vi "PDF Welding.vi"(0 "configuration file path":path caption="配置文件的路径", 1 "PDF Welding msic inf":T1) -> ()   [LabVIEW 2014]
uses:
  Ctl.xio/PDF Welding msic ctl.ctl
  SubVIS.xio/DataSocket/DataSocket_Tags.ctl
  Ctl.xio/part type.ctl
  SubVIS.xio/Creat Write List VI's/DefCtrl/Station.ctl
  SubVIS.xio/DataSocket/Write PLC Vars/Write Bool Var in.vi
  <vilib>/Utility/file.llb/Read From Spreadsheet File (string).vi
  SubVIS.xio/DataSocket/Write PLC Vars/Write String Var in.vi
  SubVIS.xio/DataSocket/Read PLC Vars/Read Bool Var.vi
  SubVIS.xio/DataSocket/Read PLC Vars/Read U32 Var.vi
  SubVIS.xio/DataSocket/Write PLC Vars/Write Dbl Var in.vi
  SubVIS.xio/Hopper car inf/Curing inf.vi
panel:
  in  "SQL information":string
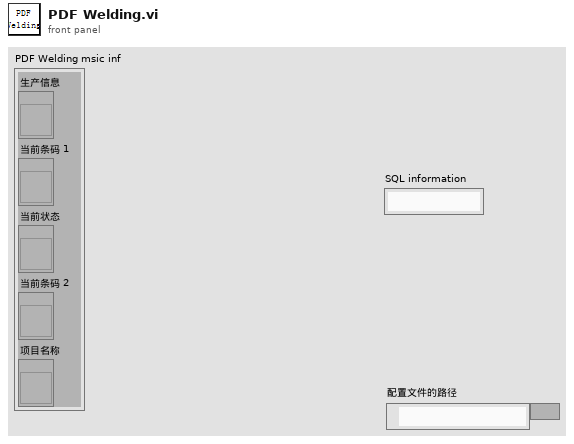
[diagram p1: front panel]
types:
  T1 = cluster{"生产信息":refnum<vi>, "当前条码 1":refnum<vi>, "当前状态":refnum<vi>, "当前条码 2":refnum<vi>, "项目名称":refnum<vi>}
  T2 = typedef "Station.ctl" = enum16{"粗切工位", "热处理工位", "精切工位", "PDF焊接工位", "打凹点预载力工位", "收卷工位", "EOL工位"}
  T3 = typedef "PDF Welding msic ctl.ctl" = cluster{"configuration file path":path, "DsOut":T4[], "Hopper car information":cluster{"Hopper car code":string, "Hopper car No":string, "plate No":string}, "pallet.produced number":i32, "SQL information":string, "Serial number":i32, "database path":path, "PDF Welding msic inf":cluster{"生产信息":refnum<vi>, "当前条码 1":refnum<vi>, "当前状态":refnum<vi>, "当前条码 2":refnum<vi>, "项目名称":refnum<vi>}, "Heating process parameters":cluster{"heating start":string, "heating finish":string, "Heating time use":u32}, "part type":T5, "Inlet temperature database":string[], "Outlet temperature database":string[], "Inlet temperature buffer":i32[], "Outlet temperature buffer":i32[], "PDF start time":string, "PDF finish time":string, "BarCode1":string, "BarCode2":string, "scanner resource name out":refnum<visa-resource-name>, "scanner coms or ip":string, "Outlet pressure buffer":i32[], "Outlet pressure database":string[], "scanner ip ID":refnum<k5>}
  T4 = typedef "DataSocket_Tags.ctl" = cluster{"Ds ID":refnum<k13>, "Tag":string}
  T5 = typedef "part type.ctl" = cluster{"项目号":string, "物料代码":string, "零件号":string, "供应商编码":string, "产线编码":string, "客户代码":string, "颜色代码":string, "托盘上限":i32, "加热温度":string, "加热时长":string, "EOL Stations":string}
  T6 = cluster{"Hopper car code":string, "Hopper car No":string, "plate No":string}
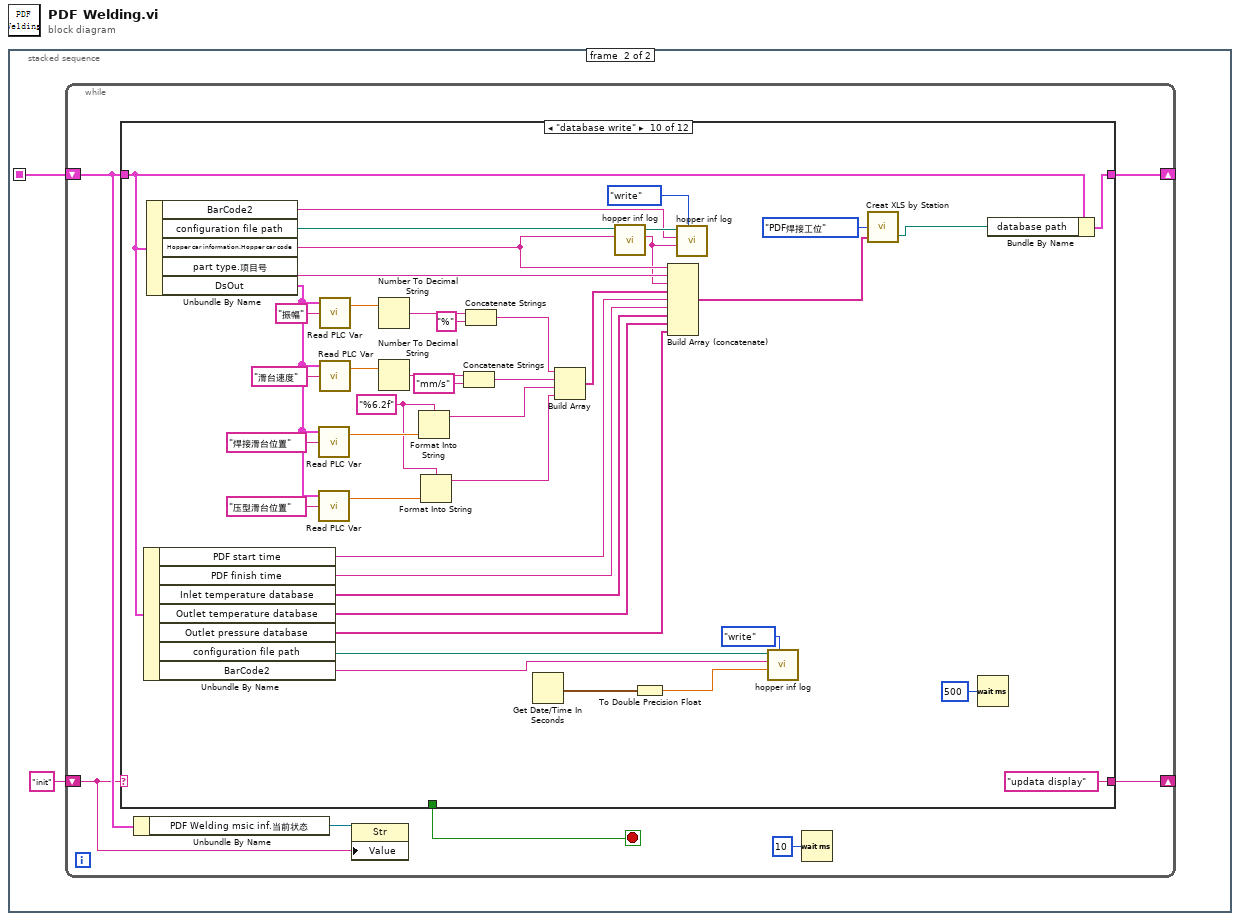
[diagram p0: block diagram]
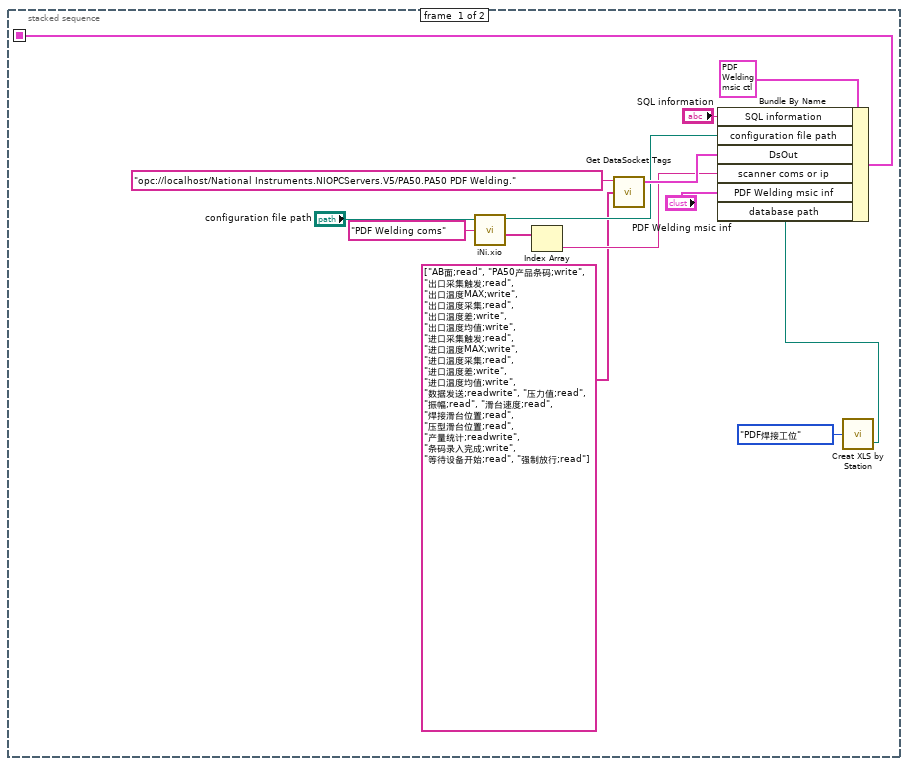
[diagram p2: hidden frame]
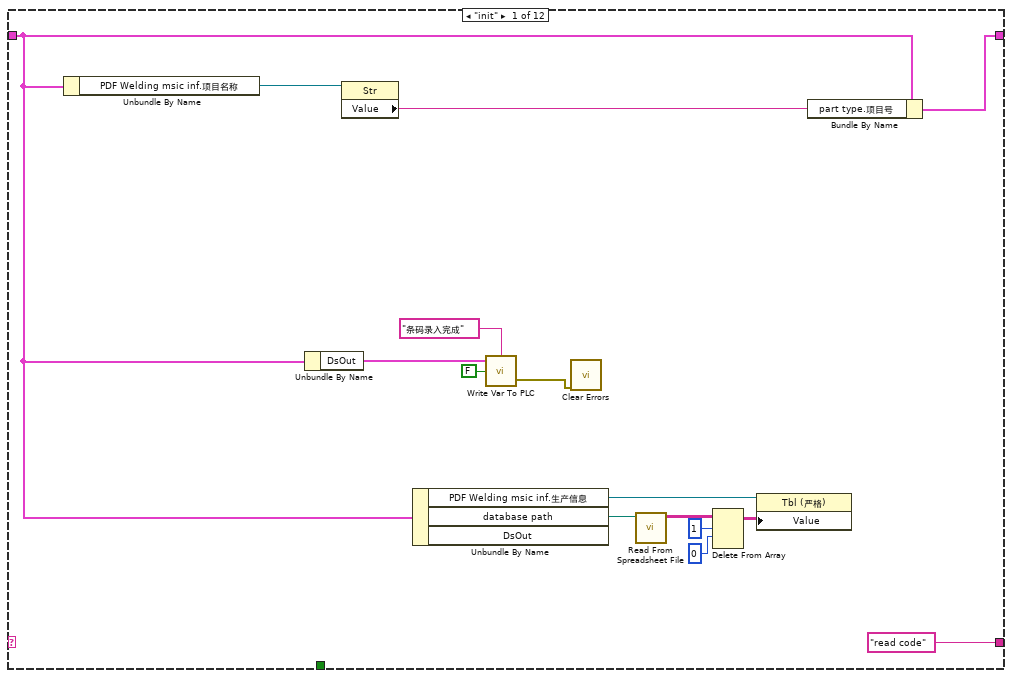
[diagram p3: hidden frame]
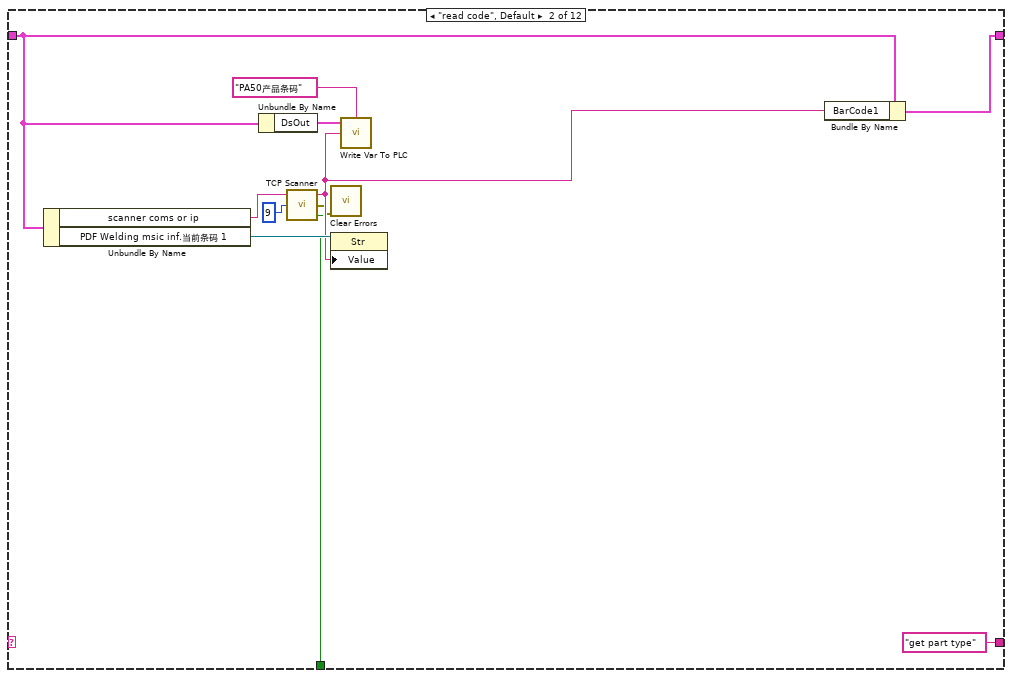
[diagram p4: hidden frame]
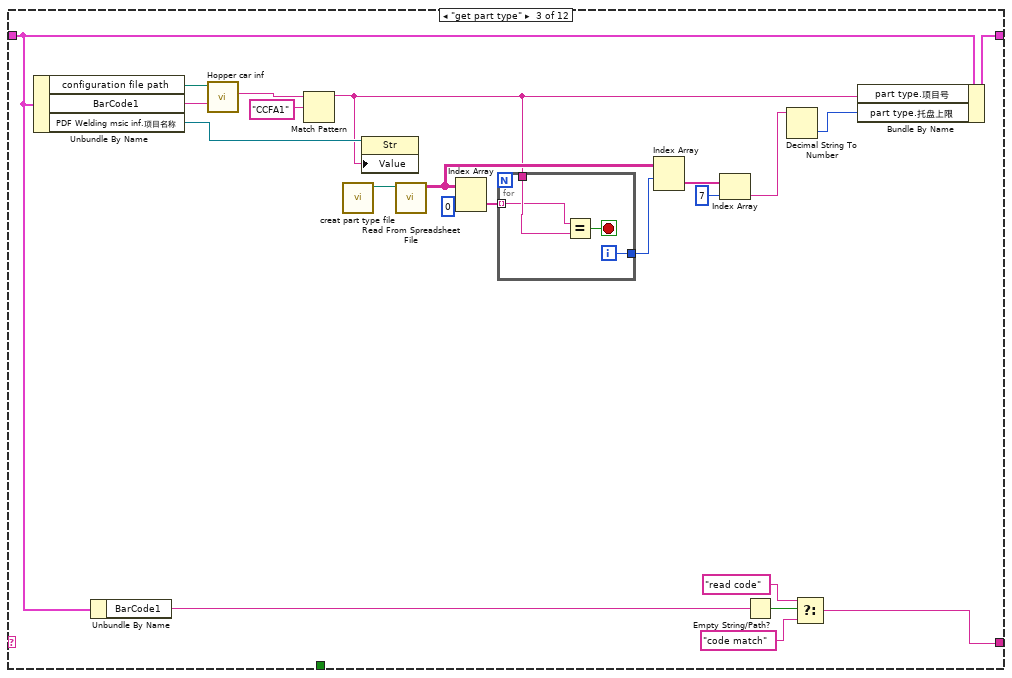
[diagram p5: hidden frame]
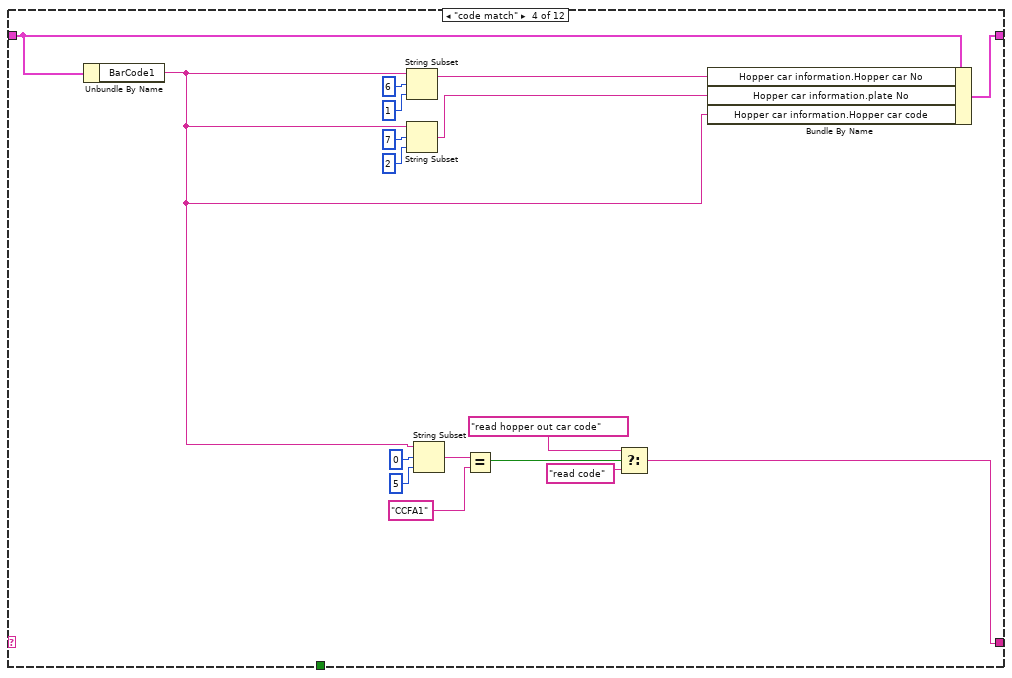
[diagram p6: hidden frame]
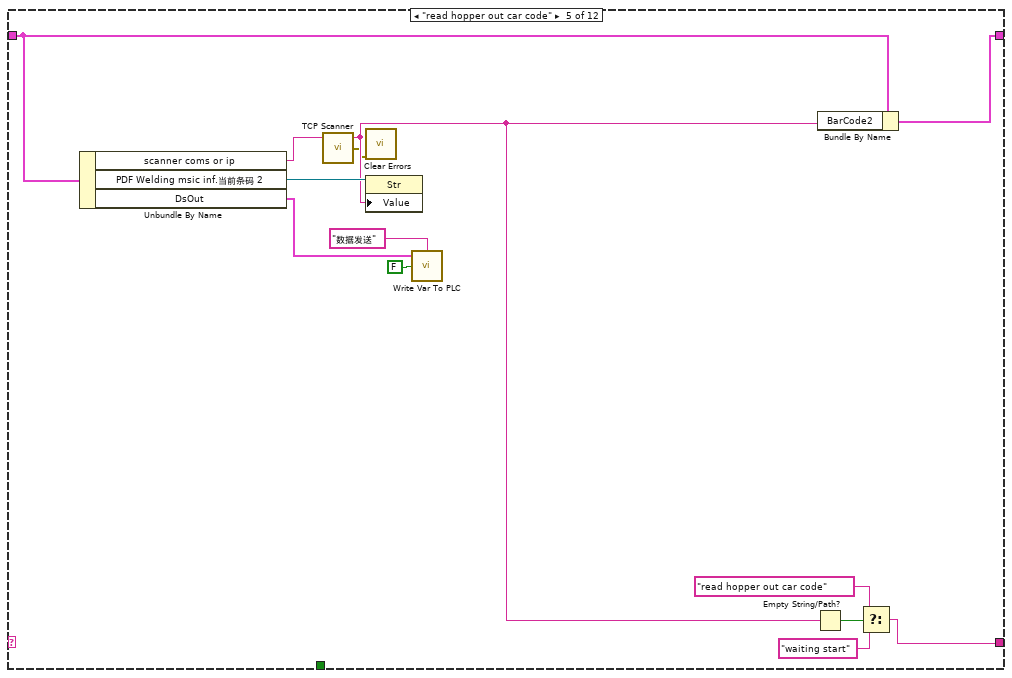
[diagram p7: hidden frame]
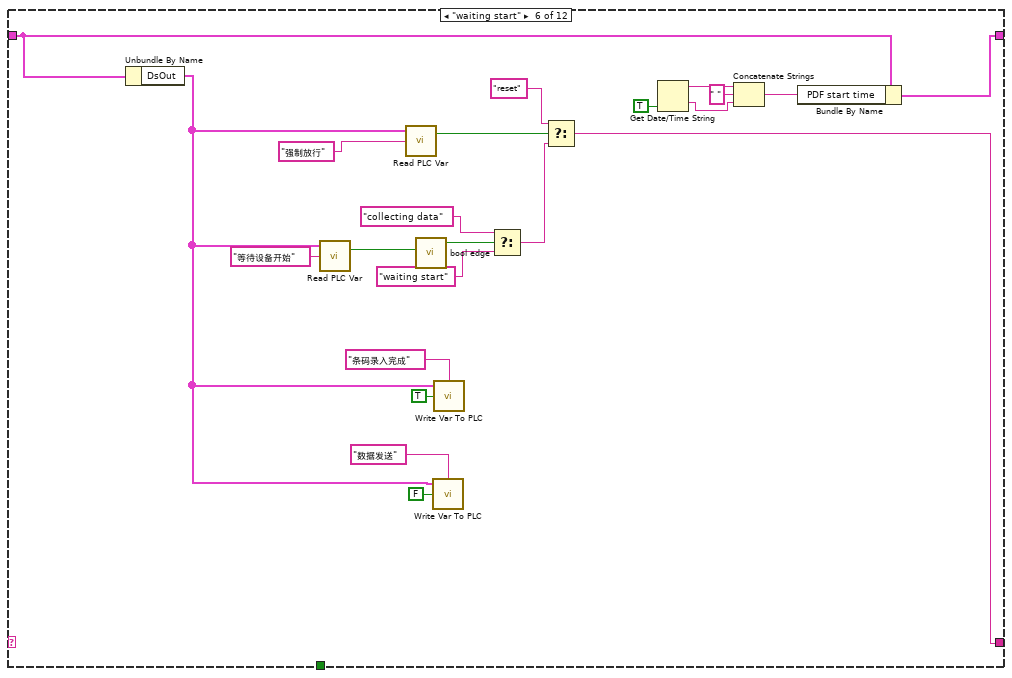
[diagram p8: hidden frame]
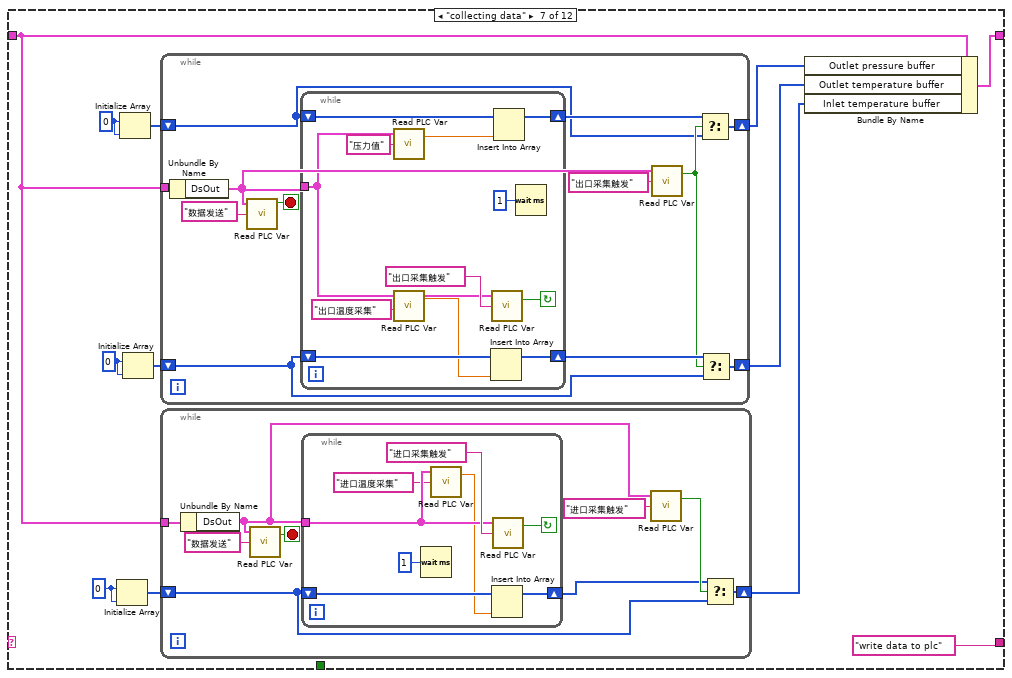
[diagram p9: hidden frame]
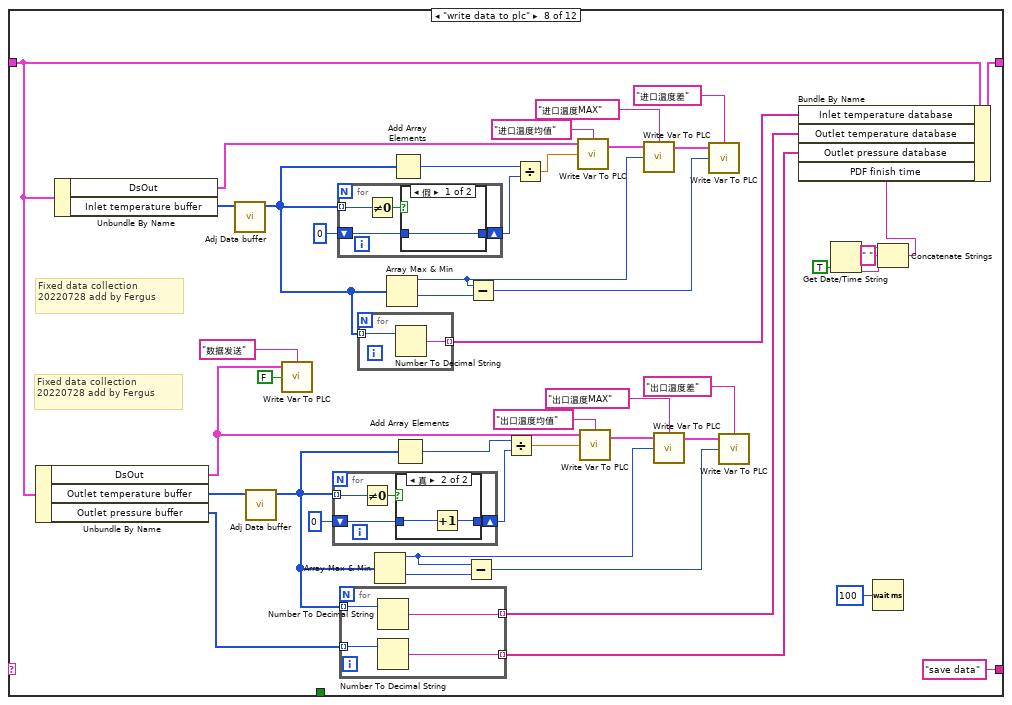
[diagram p10: hidden frame]
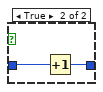
[diagram p12: hidden frame]
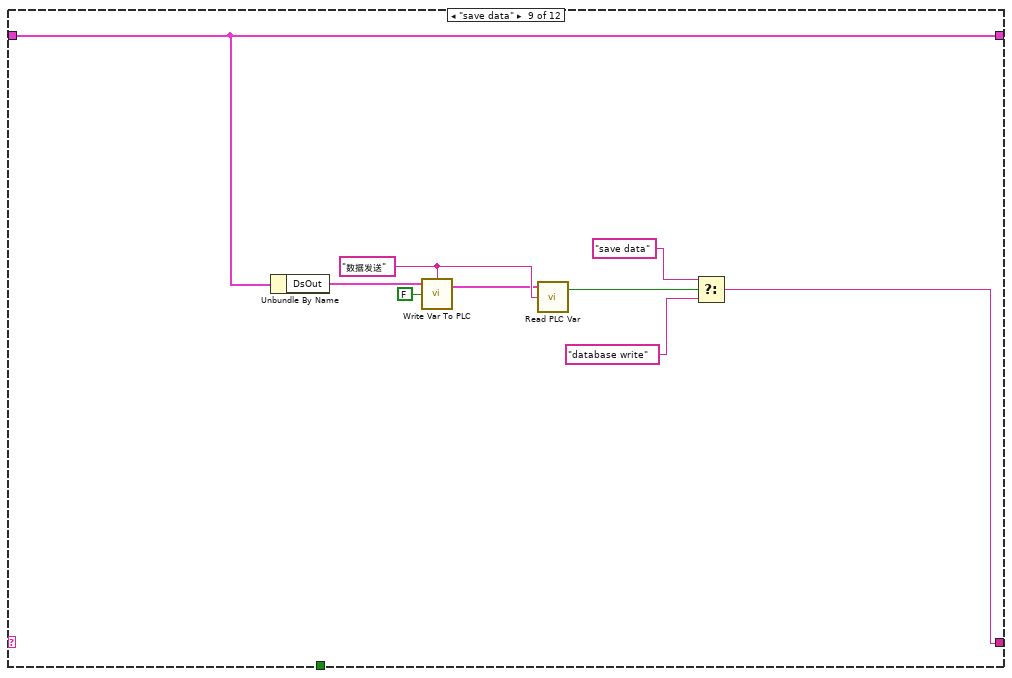
[diagram p13: hidden frame]
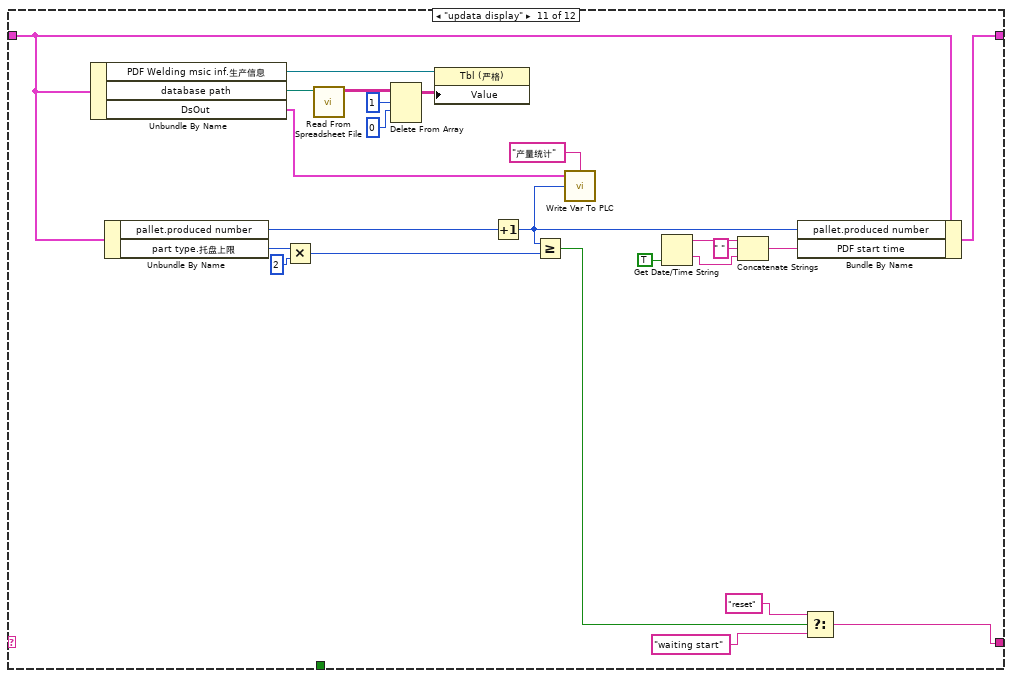
[diagram p14: hidden frame]
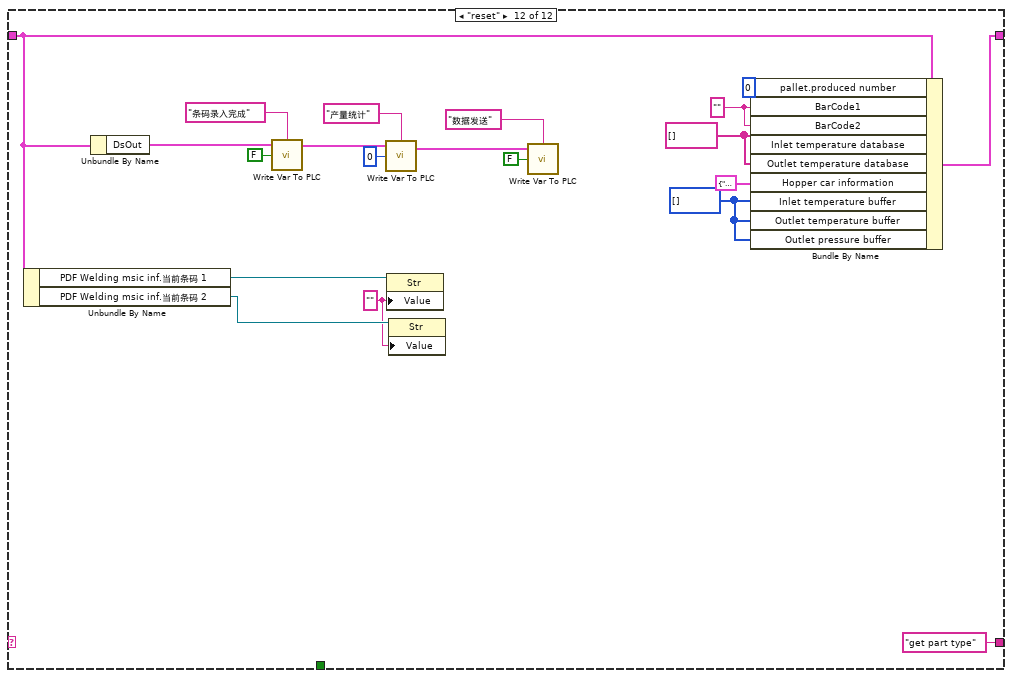
[diagram p15: hidden frame]
diagram:
  n1 = stacked-sequence {
    seq-local: [w3 _] -> [_ w15]
    frame #0 {
      n2 = call "iNi.xio.vi"("configuration file path"="configuration file path", "Sections"="PDF Welding coms") -> ("configuration file path"=w13:path, "Values"=w11:string[])  [unwired: 1 in, 3 out]
      n3 = Index Array(array=w11) -> (element=w10:string)  [unwired: 1 in]
      n4 = call "Get DataSocket Tags.vi"("All Tags"=string[] ["AB面;read", "PA50产品条码;write", "出口采集触发;read", "出口温度MAX;write", "出口温度采集;read", "出口温度差;write", "出口温度均值;write", "进口采集触发;read", "进口温度MAX;write", "进口温度采集;read", "进口温度差;write", "进口温度均值;write", "数据发送;readwrite", "压力值;read", "振幅;read", "滑台速度;read", "焊接滑台位置;read", "压型滑台位置;read", "产量统计;readwrite", "条码录入完成;write", "等待设备开始;read", "强制放行;read"], "URL"="opc://localhost/National Instruments.NIOPCServers.V5/PA50.PA50 PDF Welding.") -> ("DsOut"=w14:T4[])  [unwired: 3 in]
      n5 = call "Creat XLS by Station.vi"("staiton"=Station."PDF焊接工位") -> ("new file path (Not A Path if cancelled)"=w1:path)  [unwired: 5 in]
      n6 = Bundle By Name(cluster=T3 {"configuration file path"=path "", "DsOut"=[], "Hopper car information"={"Hopper car code"="", "Hopper car No"="", "plate No"=""}, "pallet.produced number"=0, "SQL information"="", "Serial number"=0, "database path"=path "", "PDF Welding msic inf"={"生产信息"=refnum, "当前条码 1"=refnum, "当前状态"=refnum, "当前条码 2"=refnum, "项目名称"=refnum}, "Heating process parameters"={"heating start"="", "heating finish"="", "Heating time use"=0}, "part type"={"项目号"="", "物料代码"="", "零件号"="", "供应商编码"="", "产线编码"="", "客户代码"="", "颜色代码"="", "托盘上限"=0, "加热温度"="", "加热时长"="", "EOL Stations"=""}, "Inlet temperature database"=[], "Outlet temperature database"=[], "Inlet temperature buffer"=[], "Outlet temperature buffer"=[], "PDF start time"="", "PDF finish time"="", "BarCode1"="", "BarCode2"="", "scanner resource name out"="", "scanner coms or ip"="", "Outlet pressure buffer"=[], "Outlet pressure database"=[], "scanner ip ID"=refnum} ("PDF Welding msic ctl"), "SQL information"="SQL information", "configuration file path"=w13, "DsOut"=w14, "scanner coms or ip"=w10, "PDF Welding msic inf"="PDF Welding msic inf", "database path"=w1) -> (w3:T3)
    }
    frame #1 {
      n7 = while {
        shift-right: [w23] -> _
        shift-left: w15 -> [w19]
        shift-right: [w22] -> _
        shift-left: "init" ("event") -> [w18]
        stop <- w17 stop-if-true
        n8 = case shown="\"database write\"" w18 {
          tunnel: w19 -> [w25 w46 w54 w78 w104 w108 w128 w196 w253 w295 w312 w331]
          tunnel: [w38 w49 w71 w86 w103 w106 w139 w197 w253 w296 w311 w340] -> w23
          tunnel: ["read code" "get part type" ("f") w58 w85 w97 w119 "write data to plc" ("f") "save data" ("f") w246 "updata display" ("f") w307 "get part type" ("f")] -> w22
          tunnel: [_ w39 _ _ _ _ _ _ _ _ _ _] -> w17
          frame "init" {
            n9 = Unbundle By Name(w25) -> ("PDF Welding msic inf.项目名称"=w37:refnum<vi>)
            n10 = Unbundle By Name(w25) -> ("DsOut"=w34:T4[])
            n11 = property class="Str"(reference=w37) -> ("Value"=w36:string)  [unwired: 1 in, 2 out]
            n12 = Unbundle By Name(w25) -> ("PDF Welding msic inf.生产信息"=w31:refnum<vi>, "database path"=w30:path)  [unwired: 1 out]
            n13 = call-poly "Write Var To PLC.vi"("Tag IN"="条码录入完成", "Bool Var in"=FALSE, "Ds PLCTags IN"=w34) -> ("error out"=w24:errorcluster)  [unwired: 1 in, 1 out]
            n14 = call <vilib>:"Clear Errors.vi"("error in (no error)"=w24) -> ()  [unwired: 5 in, 2 out]
            n15 = call-poly <vilib>:"Read From Spreadsheet File.vi"("file path (dialog if empty)"=w30) -> ("all rows"=w29:string[][])  [unwired: 6 in, 4 out]
            n16 = Delete From Array(array=w29, length=1 ("长度"), index (row)=0 ("索引 (行)")) -> (array with subset deleted=w26:string[][])  [unwired: 1 in, 1 out]
            n17 = property class="Tbl (严格)"(reference=w31, "Value"=w26) -> ()  [unwired: 1 in, 2 out]
            n18 = Bundle By Name(cluster=w25, "part type.项目号"=w36) -> (w38:T3)
          }
          frame "read code", Default {
            n19 = Unbundle By Name(w46) -> ("scanner coms or ip"=w42:string, "PDF Welding msic inf.当前条码 1"=w48:refnum<vi>)
            n20 = Unbundle By Name(w46) -> ("DsOut"=w45:T4[])
            n21 = call "TCP Scanner.vi"("byte of read(9)"=9 ("读取的字节"), "ip"=w42) -> ("status"=w39:bool, "错误输出"=w40:errorcluster, "Barcode"=w44:string)  [unwired: 1 in]
            n22 = call <vilib>:"Clear Errors.vi"("error in (no error)"=w40) -> ()  [unwired: 5 in, 2 out]
            n23 = property class="Str"(reference=w48, "Value"=w44) -> ()  [unwired: 1 in, 2 out]
            n24 = call-poly "Write Var To PLC.vi"("Tag IN"="PA50产品条码", "String Var in"=w44, "Ds PLCTags IN"=w45) -> ()  [unwired: 1 in, 2 out]
            n25 = Bundle By Name(cluster=w46, "BarCode1"=w44) -> (w49:T3)
          }
          frame "get part type" {
            n26 = Unbundle By Name(w54) -> ("configuration file path"=w56:path, "BarCode1"=w55:string, "PDF Welding msic inf.项目名称"=w53:refnum<vi>)
            n27 = Unbundle By Name(w54) -> ("BarCode1"=w57:string)
            n28 = call "Hopper car inf.vi"("key"=w55, "path in"=w56) -> ("value out"=w52:string)  [unwired: 8 in, 1 out]
            n29 = Match Pattern(string=w52, regular expression="CCFA1" ("正则表达式")) -> (before substring=w50:string)  [unwired: 1 in, 3 out]
            n30 = call "creat part type file.vi"() -> ("new file path (Not A Path if cancelled)"=w62:path)  [unwired: 11 in]
            n31 = property class="Str"(reference=w53, "Value"=w50) -> ()  [unwired: 1 in, 2 out]
            n32 = call-poly <vilib>:"Read From Spreadsheet File.vi"("file path (dialog if empty)"=w62) -> ("all rows"=w67:string[][])  [unwired: 6 in, 4 out]
            n33 = Index Array(array=w67, index (col)=0 ("禁用的索引 (列)")) -> (element=w69:string[])  [unwired: 1 in]
            n34 = for {
              tunnel: w69 -> [w72] mode=indexing
              tunnel: [w74] -> w66
              tunnel: w50 -> [w73]
              i -> [w74]
              stop <- w75 stop-if-true
              n35 = Equal?(x=w72, y=w73) -> (x = y?=w75:bool)
            }
            n36 = Index Array(array=w67, index (row)=w66) -> (element=w65:string[])  [unwired: 1 in]
            n37 = Index Array(array=w65, index=7 ("索引")) -> (element=w64:string)
            n38 = Empty String/Path?(string/path=w57) -> (empty?=w61:bool)
            n39 = Decimal String To Number(string=w64) -> (number=w63:i32)  [unwired: 2 in, 1 out]
            n40 = Select(t="read code", s=w61, f="code match") -> (s? t:f=w58:string)
            n41 = Bundle By Name(cluster=w54, "part type.项目号"=w50, "part type.托盘上限"=w63) -> (w71:T3)
          }
          frame "code match" {
            n42 = Unbundle By Name(w78) -> ("BarCode1"=w77:string)
            n43 = String Subset(string=w77, offset (0)=6 ("偏移量(0)"), length (rest)=1 ("长度（剩余）")) -> (substring=w80:string)
            n44 = String Subset(string=w77, offset (0)=7 ("偏移量(0)"), length (rest)=2 ("长度（剩余）")) -> (substring=w81:string)
            n45 = String Subset(string=w77, offset (0)=0 ("偏移量(0)"), length (rest)=5 ("长度（剩余）")) -> (substring=w82:string)
            n46 = Equal?(x=w82, y="CCFA1") -> (x = y?=w76:bool)
            n47 = Select(t="read hopper out car code" ("event"), s=w76, f="read code" ("event")) -> (s? t:f=w85:string)
            n48 = Bundle By Name(cluster=w78, "Hopper car information.Hopper car No"=w80, "Hopper car information.plate No"=w81, "Hopper car information.Hopper car code"=w77) -> (w86:T3)
          }
          frame "read hopper out car code" {
            n49 = Unbundle By Name(w104) -> ("scanner coms or ip"=w105:string, "PDF Welding msic inf.当前条码 2"=w102:refnum<vi>, "DsOut"=w93:T4[])
            n50 = call "TCP Scanner.vi"("ip"=w105) -> ("错误输出"=w96:errorcluster, "Barcode"=w98:string)  [unwired: 2 in, 1 out]
            n51 = call <vilib>:"Clear Errors.vi"("error in (no error)"=w96) -> ()  [unwired: 5 in, 2 out]
            n52 = property class="Str"(reference=w102, "Value"=w98) -> ()  [unwired: 1 in, 2 out]
            n53 = call-poly "Write Var To PLC.vi"("Tag IN"="数据发送", "Bool Var in"=FALSE, "Ds PLCTags IN"=w93) -> ()  [unwired: 1 in, 2 out]
            n54 = Empty String/Path?(string/path=w98) -> (empty?=w101:bool)
            n55 = Bundle By Name(cluster=w104, "BarCode2"=w98) -> (w103:T3)
            n56 = Select(t="read hopper out car code" ("f"), s=w101, f="waiting start") -> (s? t:f=w97:string)
          }
          frame "waiting start" {
            n57 = Unbundle By Name(w108) -> ("DsOut"=w113:T4[])
            n58 = call-poly "Read PLC Var.vi"("Tag IN"="等待设备开始", "Ds PLCTags IN"=w113) -> ("Bool Var out"=w126:bool)  [unwired: 1 in, 1 out]
            n59 = call-poly "Read PLC Var.vi"("Tag IN"="强制放行", "Ds PLCTags IN"=w113) -> ("Bool Var out"=w121:bool)  [unwired: 1 in, 1 out]
            n60 = call "bool edge.vi"("bool in"=w126) -> ("false-true"=w125:bool)  [unwired: 6 in, 1 out]
            n61 = call-poly "Write Var To PLC.vi"("Tag IN"="数据发送", "Bool Var in"=FALSE, "Ds PLCTags IN"=w113) -> ()  [unwired: 1 in, 2 out]
            n62 = call-poly "Write Var To PLC.vi"("Tag IN"="条码录入完成", "Bool Var in"=TRUE, "Ds PLCTags IN"=w113) -> ()  [unwired: 1 in, 2 out]
            n63 = Select(t="collecting data" ("f"), s=w125, f="waiting start") -> (s? t:f=w120:string)
            n64 = Select(t="reset" ("f"), s=w121, f=w120) -> (s? t:f=w119:string)
            n65 = Get Date/Time String(want seconds? (F)=TRUE ("需要秒？(F)")) -> (date string=w112:string, time string=w110:string)  [unwired: 2 in]
            n66 = Concatenate Strings(w112, " " ("字符串"), w110) -> (w107:string)
            n67 = Bundle By Name(cluster=w108, "PDF start time"=w107) -> (w106:T3)
          }
          frame "collecting data" {
            w131 = 0 ("维数大小")
            w133 = 0 ("维数大小")
            w136 = 0 ("维数大小")
            n68 = Initialize Array(w133, w133) -> (w132:i32[])
            n69 = Initialize Array(w131, w131) -> (w130:i32[])
            n70 = Initialize Array(w136, w136) -> (w135:i32[])
            n71 = while {
              tunnel: w128 -> [w168]
              shift-right: [w161] -> w134
              shift-left: w135 -> [w162]
              shift-right: [w160] -> w129
              shift-left: w130 -> [w157]
              stop <- w166 stop-if-true
              n72 = Unbundle By Name(w168) -> ("DsOut"=w165:T4[])
              n73 = call-poly "Read PLC Var.vi"("Tag IN"="数据发送", "Ds PLCTags IN"=w165) -> ("Bool Var out"=w166:bool)  [unwired: 1 in, 1 out]
              n74 = while {
                tunnel: w165 -> [w173]
                shift-right: [w175] -> w163
                shift-left: w162 -> [w177]
                shift-right: [w169] -> w158
                shift-left: w157 -> [w170]
                stop <- w180 continue-if-true
                n75 = call-poly "Read PLC Var.vi"("Tag IN"="压力值", "Ds PLCTags IN"=w173) -> ("U32 Var out"=w171:dbl)  [unwired: 1 in, 1 out]
                n76 = call-poly "Read PLC Var.vi"("Tag IN"="出口温度采集", "Ds PLCTags IN"=w173) -> ("U32 Var out"=w176:dbl)  [unwired: 1 in, 1 out]
                n77 = Insert Into Array(array=w177, new element=w176) -> (w175:i32[])  [unwired: 1 in]
                n78 = call-poly "Read PLC Var.vi"("Tag IN"="出口采集触发", "Ds PLCTags IN"=w173) -> ("Bool Var out"=w180:bool)  [unwired: 1 in, 1 out]
                n79 = Insert Into Array(array=w170, new element=w171) -> (w169:i32[])  [unwired: 1 in]
                n80 = Wait (ms)(milliseconds to wait=u32 1 ("等待时间（毫秒）")) -> ()  [unwired: 1 out]
              }
              n81 = call-poly "Read PLC Var.vi"("Tag IN"="出口采集触发", "Ds PLCTags IN"=w165) -> ("Bool Var out"=w159:bool)  [unwired: 1 in, 1 out]
              n82 = Select(t=w158, s=w159, f=w157) -> (s? t:f=w160:i32[])
              n83 = Select(t=w163, s=w159, f=w162) -> (s? t:f=w161:i32[])
            }
            n84 = while {
              tunnel: w128 -> [w148]
              shift-right: [w143] -> w138
              shift-left: w132 -> [w140]
              stop <- w146 stop-if-true
              n85 = Unbundle By Name(w148) -> ("DsOut"=w145:T4[])
              n86 = call-poly "Read PLC Var.vi"("Tag IN"="数据发送", "Ds PLCTags IN"=w145) -> ("Bool Var out"=w146:bool)  [unwired: 1 in, 1 out]
              n87 = while {
                tunnel: w145 -> [w154]
                shift-right: [w150] -> w141
                shift-left: w140 -> [w152]
                stop <- w156 continue-if-true
                n88 = Wait (ms)(milliseconds to wait=u32 1 ("等待时间（毫秒）")) -> ()  [unwired: 1 out]
                n89 = call-poly "Read PLC Var.vi"("Tag IN"="进口温度采集", "Ds PLCTags IN"=w154) -> ("U32 Var out"=w151:dbl)  [unwired: 1 in, 1 out]
                n90 = Insert Into Array(array=w152, new element=w151) -> (w150:i32[])  [unwired: 1 in]
                n91 = call-poly "Read PLC Var.vi"("Tag IN"="进口采集触发", "Ds PLCTags IN"=w154) -> ("Bool Var out"=w156:bool)  [unwired: 1 in, 1 out]
              }
              n92 = call-poly "Read PLC Var.vi"("Tag IN"="进口采集触发", "Ds PLCTags IN"=w145) -> ("Bool Var out"=w142:bool)  [unwired: 1 in, 1 out]
              n93 = Select(t=w141, s=w142, f=w140) -> (s? t:f=w143:i32[])
            }
            n94 = Bundle By Name(cluster=w128, "Outlet pressure buffer"=w129, "Outlet temperature buffer"=w134, "Inlet temperature buffer"=w138) -> (w139:T3)
          }
          frame "write data to plc" {
            # "Fixed data collection\n20220728 add by Fergus"
            # "Fixed data collection\n20220728 add by Fergus"
            n95 = Unbundle By Name(w196) -> ("DsOut"=w193:T4[], "Outlet temperature buffer"=w182:i32[], "Outlet pressure buffer"=w187:i32[])
            n96 = Unbundle By Name(w196) -> ("DsOut"=w221:T4[], "Inlet temperature buffer"=w184:i32[])
            n97 = call "Adj Data buffer.vi"("data buffer"=w184) -> ("data buffer out"=w183:i32[])  [unwired: 10 in]
            n98 = call "Adj Data buffer.vi"("data buffer"=w182) -> ("data buffer out"=w181:i32[])  [unwired: 10 in]
            n99 = call-poly "Write Var To PLC.vi"("Tag IN"="数据发送", "Bool Var in"=FALSE, "Ds PLCTags IN"=w193) -> ()  [unwired: 1 in, 2 out]
            n100 = for {
              tunnel: w181 -> [w235] mode=indexing
              shift-right: [w232] -> w216
              shift-left: 0 -> [w233]
              n101 = Not Equal To 0?(x=w235) -> (x != 0?=w234:bool)
              n102 = case shown="真" w234 {
                tunnel: w233 -> [w236 w237]
                tunnel: [w236 w238] -> w232
                frame False {
                }
                frame True {
                  n103 = Increment(x=w237) -> (x+1=w238:i32)
                }
              }
            }
            n104 = for {
              tunnel: w183 -> [w242] mode=indexing
              shift-right: [w239] -> w223
              shift-left: 0 -> [w240]
              n105 = Not Equal To 0?(x=w242) -> (x != 0?=w241:bool)
              n106 = case shown="假" w241 {
                tunnel: w240 -> [w243 w244]
                tunnel: [w243 w245] -> w239
                frame False {
                }
                frame True {
                  n107 = Increment(x=w244) -> (x+1=w245:i32)
                }
              }
            }
            n108 = for {
              tunnel: w181 -> [w229] mode=indexing
              tunnel: [w227] -> w199 mode=indexing
              tunnel: w187 -> [w228] mode=indexing
              tunnel: [w226] -> w185 mode=indexing
              n109 = Number To Decimal String(number=w229) -> (decimal integer string=w227:string)  [unwired: 1 in]
              n110 = Number To Decimal String(number=w228) -> (decimal integer string=w226:string)  [unwired: 1 in]
            }
            n111 = for {
              tunnel: w183 -> [w231] mode=indexing
              tunnel: [w230] -> w200 mode=indexing
              n112 = Number To Decimal String(number=w231) -> (decimal integer string=w230:string)  [unwired: 1 in]
            }
            n113 = Array Max & Min(array=w181) -> (max value=w203:i32, min value=w202:i32)  [unwired: 2 out]
            n114 = Array Max & Min(array=w183) -> (max value=w211:i32, min value=w214:i32)  [unwired: 2 out]
            n115 = Add Array Elements(numeric array=w183) -> (sum=w222:i32)
            n116 = Add Array Elements(numeric array=w181) -> (sum=w217:i32)
            n117 = Subtract(x=w203, y=w202) -> (x-y=w201:i32)
            n118 = Subtract(x=w211, y=w214) -> (x-y=w208:i32)
            n119 = Divide(x=w217, y=w216) -> (x/y=w215:dbl)
            n120 = Divide(x=w222, y=w223) -> (x/y=w219:dbl)
            n121 = call-poly "Write Var To PLC.vi"("Tag IN"="进口温度均值", "Dbl Var in"=w219, "Ds PLCTags IN"=w221) -> ("Ds PLCTags OUT"=w213:T4[])  [unwired: 1 in, 1 out]
            n122 = call-poly "Write Var To PLC.vi"("Tag IN"="出口温度均值", "Dbl Var in"=w215, "Ds PLCTags IN"=w193) -> ("Ds PLCTags OUT"=w204:T4[])  [unwired: 1 in, 1 out]
            n123 = call-poly "Write Var To PLC.vi"("Tag IN"="进口温度MAX", "Dbl Var in"=w211, "Ds PLCTags IN"=w213) -> ("Ds PLCTags OUT"=w210:T4[])  [unwired: 1 in, 1 out]
            n124 = call-poly "Write Var To PLC.vi"("Tag IN"="出口温度MAX", "Dbl Var in"=w203, "Ds PLCTags IN"=w204) -> ("Ds PLCTags OUT"=w206:T4[])  [unwired: 1 in, 1 out]
            n125 = call-poly "Write Var To PLC.vi"("Tag IN"="进口温度差", "Dbl Var in"=w208, "Ds PLCTags IN"=w210) -> ()  [unwired: 1 in, 2 out]
            n126 = call-poly "Write Var To PLC.vi"("Tag IN"="出口温度差", "Dbl Var in"=w201, "Ds PLCTags IN"=w206) -> ()  [unwired: 1 in, 2 out]
            n127 = Get Date/Time String(want seconds? (F)=TRUE ("需要秒？(F)")) -> (date string=w192:string, time string=w190:string)  [unwired: 2 in]
            n128 = Wait (ms)(milliseconds to wait=u32 100 ("等待时间（毫秒）")) -> ()  [unwired: 1 out]
            n129 = Concatenate Strings(w192, " " ("字符串"), w190) -> (w188:string)
            n130 = Bundle By Name(cluster=w196, "Inlet temperature database"=w200, "Outlet temperature database"=w199, "Outlet pressure database"=w185, "PDF finish time"=w188) -> (w197:T3)
          }
          frame "save data" {
            w251 = "数据发送" ("Tag IN")
            n131 = Unbundle By Name(w253) -> ("DsOut"=w252:T4[])
            n132 = call-poly "Write Var To PLC.vi"("Tag IN"=w251, "Bool Var in"=FALSE, "Ds PLCTags IN"=w252) -> ("Ds PLCTags OUT"=w250:T4[])  [unwired: 1 in, 1 out]
            n133 = call-poly "Read PLC Var.vi"("Tag IN"=w251, "Ds PLCTags IN"=w250) -> ("Bool Var out"=w249:bool)  [unwired: 1 in, 1 out]
            n134 = Select(t="save data" ("f"), s=w249, f="database write") -> (s? t:f=w246:string)
          }
          frame "database write" {
            w261 = "%6.2f" ("格式字符串")
            n135 = Unbundle By Name(w295) -> ("PDF start time"=w291:string, "PDF finish time"=w290:string, "Inlet temperature database"=w289:string[], "Outlet temperature database"=w288:string[], "Outlet pressure database"=w258:string[], "configuration file path"=w278:path, "BarCode2"=w275:string)
            n136 = Unbundle By Name(w295) -> ("BarCode2"=w285:string, "configuration file path"=w294:path, "Hopper car information.Hopper car code"=w293:string, "part type.项目号"=w292:string, "DsOut"=w284:T4[])
            n137 = call-poly "Read PLC Var.vi"("Tag IN"="焊接滑台位置", "Ds PLCTags IN"=w284) -> ("U32 Var out"=w264:dbl)  [unwired: 1 in, 1 out]
            n138 = call-poly "Read PLC Var.vi"("Tag IN"="压型滑台位置", "Ds PLCTags IN"=w284) -> ("U32 Var out"=w262:dbl)  [unwired: 1 in, 1 out]
            n139 = call-poly "Read PLC Var.vi"("Tag IN"="振幅", "Ds PLCTags IN"=w284) -> ("U32 Var out"=w273:dbl)  [unwired: 1 in, 1 out]
            n140 = call-poly "Read PLC Var.vi"("Tag IN"="滑台速度", "Ds PLCTags IN"=w284) -> ("U32 Var out"=w270:dbl)  [unwired: 1 in, 1 out]
            n141 = Number To Decimal String(number=w273) -> (decimal integer string=w272:string)  [unwired: 1 in]
            n142 = Number To Decimal String(number=w270) -> (decimal integer string=w269:string)  [unwired: 1 in]
            n143 = Format Into String(format string=w261, w264) -> (resulting string=w263:string)  [unwired: 2 in, 1 out]
            n144 = Format Into String(format string=w261, w262) -> (resulting string=w260:string)  [unwired: 2 in, 1 out]
            n145 = Concatenate Strings(w269, "mm/s" ("字符串")) -> (w266:string)
            n146 = Concatenate Strings(w272, "%" ("字符串")) -> (w267:string)
            n147 = Get Date/Time In Seconds() -> (seconds since 1Jan1904=w277:timestamp)
            n148 = Build Array(w267, w266, w263, w260) -> (w265:string[])
            n149 = call-poly "hopper inf log.vi"("key"=w293, "path in"=w294) -> ("value out"=w279:string, "path out"=w287:path)  [unwired: 8 in]
            n150 = To Double Precision Float(number=w277) -> (double precision float=w276:dbl)
            n151 = Build Array (concatenate)(w293, w292, w279, w265, w291, w290, w289, w288, w258) -> (w255:string[])
            n152 = call-poly "hopper inf log.vi"("write\\read（read)"=enum16{"read", "write"}."write" ("write\\read（read)"), "value"=w279, "key"=w285, "path in"=w287) -> ()  [unwired: 6 in, 2 out]
            n153 = call-poly "hopper inf log.vi"("write\\read（read)"=enum16{"read", "write"}."write" ("write\\read（read)"), "value in"=w276, "key"=w275, "path in"=w278) -> ()  [unwired: 6 in, 2 out]
            n154 = call "Creat XLS by Station.vi"("staiton"=Station."PDF焊接工位", "data in"=w255) -> ("new file path (Not A Path if cancelled)"=w256:path)  [unwired: 4 in]
            n155 = Wait (ms)(milliseconds to wait=u32 500 ("等待时间（毫秒）")) -> ()  [unwired: 1 out]
            n156 = Bundle By Name(cluster=w295, "database path"=w256) -> (w296:T3)
          }
          frame "updata display" {
            n157 = Unbundle By Name(w312) -> ("PDF Welding msic inf.生产信息"=w321:refnum<vi>, "database path"=w320:path, "DsOut"=w305:T4[])
            n158 = Unbundle By Name(w312) -> ("pallet.produced number"=w306:i32, "part type.托盘上限"=w315:i32)
            n159 = Multiply(x=w315, y=2) -> (x*y=w313:i32)
            n160 = call-poly <vilib>:"Read From Spreadsheet File.vi"("file path (dialog if empty)"=w320) -> ("all rows"=w319:string[][])  [unwired: 6 in, 4 out]
            n161 = Delete From Array(array=w319, length=1 ("长度"), index (row)=0 ("索引 (行)")) -> (array with subset deleted=w316:string[][])  [unwired: 1 in, 1 out]
            n162 = property class="Tbl (严格)"(reference=w321, "Value"=w316) -> ()  [unwired: 1 in, 2 out]
            n163 = Increment(x=w306) -> (x+1=w303:i32)
            n164 = Greater Or Equal?(x=w303, y=w313) -> (x >= y?=w310:bool)
            n165 = call-poly "Write Var To PLC.vi"("Tag IN"="产量统计", "Dbl Var in"=w303, "Ds PLCTags IN"=w305) -> ()  [unwired: 1 in, 2 out]
            n166 = Get Date/Time String(want seconds? (F)=TRUE ("需要秒？(F)")) -> (date string=w302:string, time string=w300:string)  [unwired: 2 in]
            n167 = Concatenate Strings(w302, " " ("字符串"), w300) -> (w298:string)
            n168 = Bundle By Name(cluster=w312, "pallet.produced number"=w303, "PDF start time"=w298) -> (w311:T3)
            n169 = Select(t="reset" ("f"), s=w310, f="waiting start") -> (s? t:f=w307:string)
          }
          frame "reset" {
            w328 = "" ("值")
            w335 = i32[] [] ("Inlet temperature buffer")
            w337 = string[] [] ("Database")
            w336 = "" ("BarCode")
            n170 = Unbundle By Name(w331) -> ("PDF Welding msic inf.当前条码 1"=w330:refnum<vi>, "PDF Welding msic inf.当前条码 2"=w329:refnum<vi>)
            n171 = Unbundle By Name(w331) -> ("DsOut"=w334:T4[])
            n172 = call-poly "Write Var To PLC.vi"("Tag IN"="条码录入完成", "Bool Var in"=FALSE, "Ds PLCTags IN"=w334) -> ("Ds PLCTags OUT"=w327:T4[])  [unwired: 1 in, 1 out]
            n173 = call-poly "Write Var To PLC.vi"("Tag IN"="产量统计", "Dbl Var in"=0, "Ds PLCTags IN"=w327) -> ("Ds PLCTags OUT"=w322:T4[])  [unwired: 1 in, 1 out]
            n174 = property class="Str"(reference=w330, "Value"=w328) -> ()  [unwired: 1 in, 2 out]
            n175 = property class="Str"(reference=w329, "Value"=w328) -> ()  [unwired: 1 in, 2 out]
            n176 = call-poly "Write Var To PLC.vi"("Tag IN"="数据发送", "Bool Var in"=FALSE, "Ds PLCTags IN"=w322) -> ()  [unwired: 1 in, 2 out]
            n177 = Bundle By Name(cluster=w331, "pallet.produced number"=0, "BarCode1"=w336, "BarCode2"=w336, "Inlet temperature database"=w337, "Outlet temperature database"=w337, "Hopper car information"=T6 {"Hopper car code"="", "Hopper car No"="", "plate No"=""}, "Inlet temperature buffer"=w335, "Outlet temperature buffer"=w335, "Outlet pressure buffer"=w335) -> (w340:T3)
          }
        }
        n178 = Unbundle By Name(w19) -> ("PDF Welding msic inf.当前状态"=w20:refnum<vi>)
        n179 = property class="Str"(reference=w20, "Value"=w18) -> ()  [unwired: 1 in, 2 out]
        n180 = Wait (ms)(milliseconds to wait=u32 10 ("等待时间（毫秒）")) -> ()  [unwired: 1 out]
      }
    }
  }
